vi "SaveBG (SubVI).vi"(7 "BG path":path, 8 "error in (no error)":errorcluster, 9 "Channel 3":cluster{"2DRawBgIn":dbl[][], "CtrlV":dbl[]}, 10 "Channel 2":cluster{"2DRawBgIn":dbl[][], "CtrlV":dbl[]}, 11 "Channel1":cluster{"2DRawBgIn":dbl[][], "CtrlV":dbl[]}) -> (0 "error out":errorcluster)   [LabVIEW 2019]
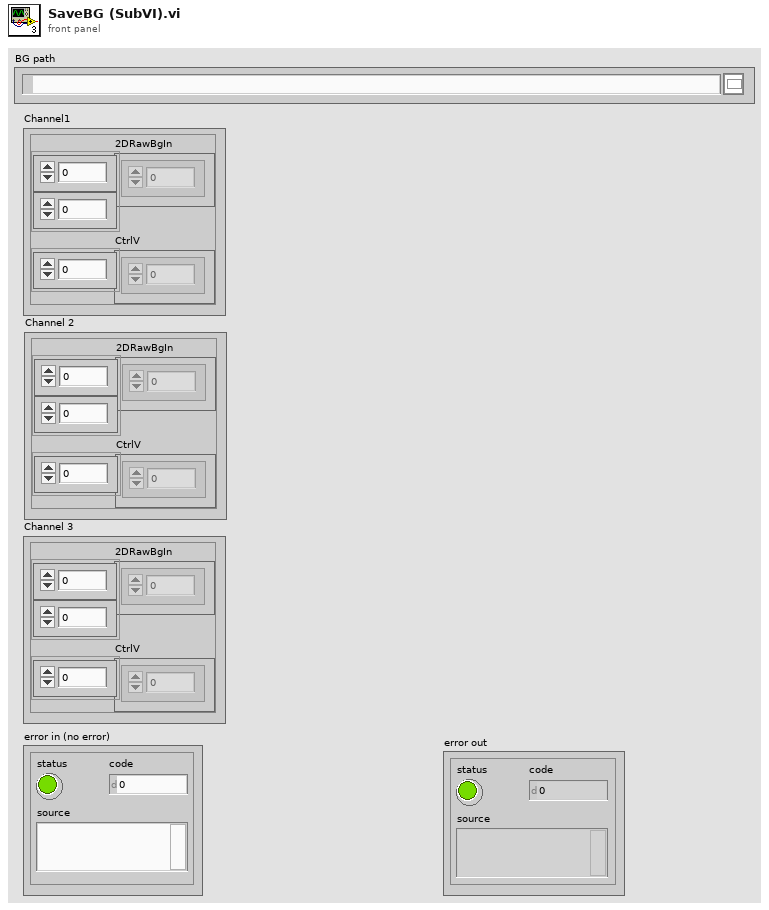
[diagram p1: front panel]
types:
  T1 = enum16{"open", "open or create", "create or replace", "create", "open (read-only)"}
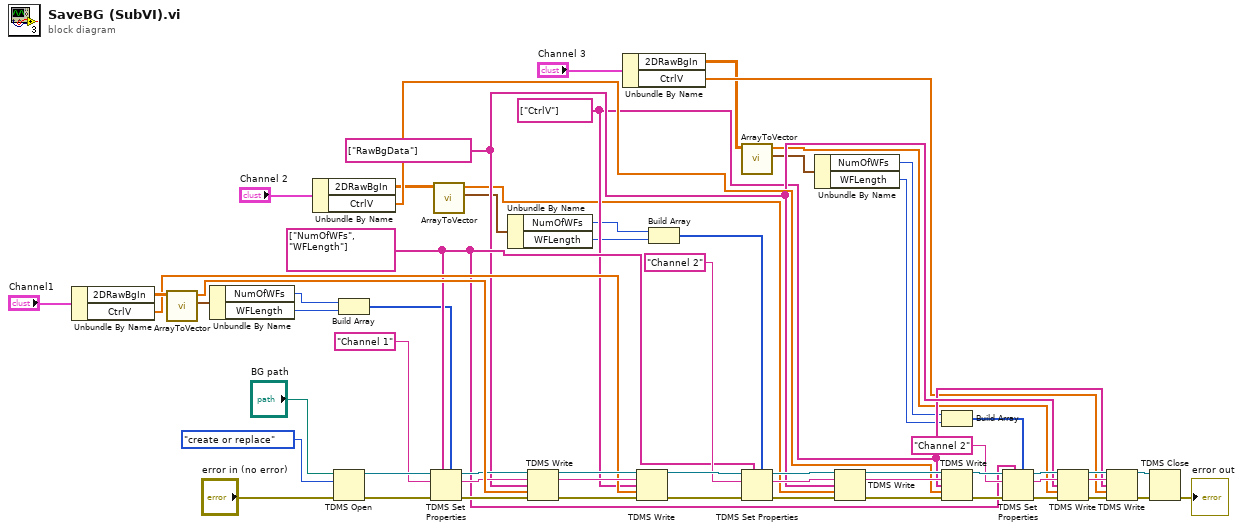
[diagram p0: block diagram]
diagram:
  w20 = string[] ["CtrlV"] ("channel name(s) in (Untitled)")
  w24 = string[] ["NumOfWFs", "WFLength"] ("property names")
  w21 = string[] ["RawBgData"] ("channel name(s) in (Untitled)")
  n1 = Unbundle By Name("Channel1") -> ("2DRawBgIn"=w52:dbl[][], "CtrlV"=w46:dbl[])
  n2 = call "ArrayToVector.vi"("2D WF in"=w52) -> ("WF Dimension"=w16:cluster{"NumOfWFs":i32, "WFLength":i32}, "1D WF out"=w53:dbl[])  [unwired: 8 in, 1 out]
  n3 = Unbundle By Name(w16) -> ("NumOfWFs"=w15:i32, "WFLength"=w14:i32)
  n4 = Unbundle By Name("Channel 2") -> ("2DRawBgIn"=w12:dbl[][], "CtrlV"=w33:dbl[])
  n5 = TDMS Open(8:"error in (no error)", 10:T1."create or replace" ("operation (0:open)"), 11:"BG path") -> (0:w56:errorcluster, 3:w57:refnum<k34>)  [unwired: 4 in]
  n6 = Build Array(w15, w14) -> (w13:i32[])
  n7 = TDMS Set Properties(5:w13, 7:w24, 8:w56, 10:"Channel 1" ("group name in (Untitled)"), 11:w57) -> (0:w50:errorcluster, 2:w39:string, 3:w51:refnum<k34>)  [unwired: 1 in, 1 out]
  n8 = call "ArrayToVector.vi"("2D WF in"=w12) -> ("WF Dimension"=w10:cluster{"NumOfWFs":i32, "WFLength":i32}, "1D WF out"=w11:dbl[])  [unwired: 8 in, 1 out]
  n9 = Unbundle By Name(w10) -> ("NumOfWFs"=w9:i32, "WFLength"=w8:i32)
  n10 = TDMS Write(0:w51, 5:w39, 7:w21, 9:w53, 11:w50) -> (4:w48:refnum<k34>, 6:w49:string, 15:w47:errorcluster)  [unwired: 1 in, 1 out]
  n11 = Unbundle By Name("Channel 3") -> ("2DRawBgIn"=w5:dbl[][], "CtrlV"=w19:dbl[])
  n12 = TDMS Write(0:w48, 5:w49, 7:w20, 9:w46, 11:w47) -> (4:w45:refnum<k34>, 15:w44:errorcluster)  [unwired: 1 in, 2 out]
  n13 = Build Array(w9, w8) -> (w7:i32[])
  n14 = call "ArrayToVector.vi"("2D WF in"=w5) -> ("WF Dimension"=w4:cluster{"NumOfWFs":i32, "WFLength":i32}, "1D WF out"=w6:dbl[])  [unwired: 8 in, 1 out]
  n15 = TDMS Set Properties(5:w7, 7:w24, 8:w44, 10:"Channel 2" ("group name in (Untitled)"), 11:w45) -> (0:w37:errorcluster, 2:w38:string, 3:w41:refnum<k34>)  [unwired: 1 in, 1 out]
  n16 = Unbundle By Name(w4) -> ("NumOfWFs"=w3:i32, "WFLength"=w2:i32)
  n17 = TDMS Write(0:w41, 5:w38, 7:w21, 9:w11, 11:w37) -> (4:w36:refnum<k34>, 6:w34:string, 15:w35:errorcluster)  [unwired: 1 in, 1 out]
  n18 = Build Array(w3, w2) -> (w1:i32[])
  n19 = TDMS Write(0:w36, 5:w34, 7:w20, 9:w33, 11:w35) -> (4:w31:refnum<k34>, 15:w30:errorcluster)  [unwired: 1 in, 2 out]
  n20 = TDMS Set Properties(5:w1, 7:w24, 8:w30, 10:"Channel 2" ("group name in (Untitled)"), 11:w31) -> (0:w28:errorcluster, 2:w23:string, 3:w29:refnum<k34>)  [unwired: 1 in, 1 out]
  n21 = TDMS Write(0:w29, 5:w23, 7:w21, 9:w6, 11:w28) -> (4:w27:refnum<k34>, 6:w22:string, 15:w26:errorcluster)  [unwired: 1 in, 1 out]
  n22 = TDMS Write(0:w27, 5:w22, 7:w20, 9:w19, 11:w26) -> (4:w18:refnum<k34>, 15:w17:errorcluster)  [unwired: 1 in, 2 out]
  n23 = TDMS Close(8:w17, 11:w18) -> (0:→"error out":errorcluster)  [unwired: 1 out]
